vi "BlockDiagram_SetInputs.vi"(7 "PythonConverter in":refnum<class "PythonBDConverter.lvclass">, 8 "error in":errorcluster, 11 "VI Interpreter in":refnum<class "VI Interpreter.lvclass">) -> (0 "error out":errorcluster, 3 "VI Interpreter out":refnum<class "VI Interpreter.lvclass">, 4 "set_inputs":string, 5 "PythonConverter out":refnum<class "PythonBDConverter.lvclass">)   [LabVIEW 2014, in "PythonBDConverter.lvclass"]
uses:
  PythonBDConverter.lvclass
  VI Interpreter/Classes/VI Interpreter/VI Interpreter.lvclass
  Parsing/ClassTypeTD.ctl
  VI Interpreter/Classes/ControlTerminal/ControlTerminal.lvclass
  VI Interpreter/Classes/TopLevelDiagram/TopLevelDiagram.lvclass
  Parsing/Python Functions.lvlib
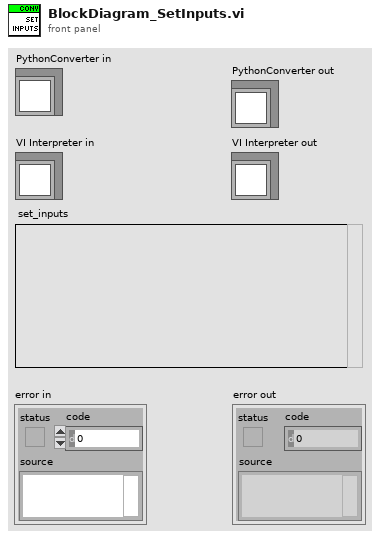
[diagram p1: front panel]
types:
  T1 = typedef "Python Functions.lvlib/ClassTypeTD.ctl" = enum16{"class", "function"}
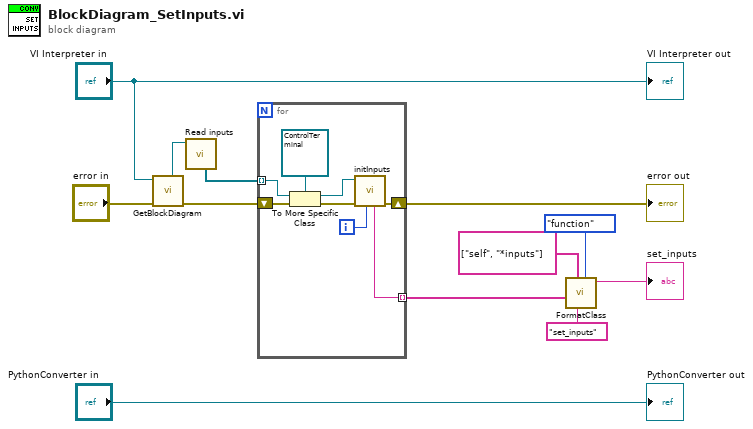
[diagram p0: block diagram]
diagram:
  n1 = call "GetBlockDiagram.vi"("error in"="error in", "VI Interpreter in"="VI Interpreter in") -> ("error out"=w5:errorcluster, "TopLevelDiagram"=w7:refnum<class "TopLevelDiagram.lvclass">)  [unwired: 5 in, 1 out]
  n2 = call-dynamic "Read inputs.vi"("Diagram in"=w7) -> ("inputs"=w6:refnum<class "Terminal.lvclass">[])  [unwired: 7 in, 1 out]
  n3 = for {
    tunnel: w6 -> [w13] mode=indexing
    shift-right: [w20] -> w4
    shift-left: w5 -> [w17]
    tunnel: [w19] -> w9 mode=indexing
    i -> [w18]
    n4 = To More Specific Class(target class=refnum<class "ControlTerminal.lvclass"> refnum ("Control Terminal in"), reference=w13, error in=w17) -> (specific class reference=w15:refnum<class "ControlTerminal.lvclass">, error out=w16:errorcluster)
    n5 = call "initInputs.vi"("index"=w18, "error in"=w16, "Control Terminal in"=w15) -> ("error out"=w20:errorcluster, "initValues"=w19:string)  [unwired: 4 in, 1 out]
  }
  "error out" <- w4
  n6 = call "FormatClass.vi"("type"=ClassTypeTD."function", "name"="set_inputs", "parameters/ancestors"=string[] ["self", "*inputs"], "body"=w9) -> ("python"=→"set_inputs":string)  [unwired: 7 in]
  "PythonConverter out" <- "PythonConverter in"
  "VI Interpreter out" <- "VI Interpreter in"
